vi "TestFGV.vi"() -> ()   [LabVIEW 2015]
uses:
  TypeDef/ActionEnum.ctl
panel:
  out "Flag Out 4":bool[](array[boolean])
  out "Flag Out 3":bool[](array[boolean])
  out "Flag Out 2":bool[](array[boolean])
  out "Flag Out":bool[](array[boolean])
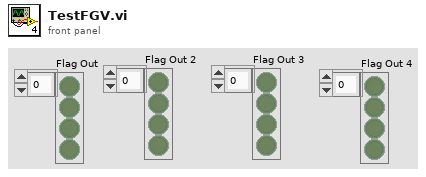
[diagram p1: front panel]
types:
  T1 = typedef "ActionEnum.ctl" = enum16{"Init", "Read", "Write"}
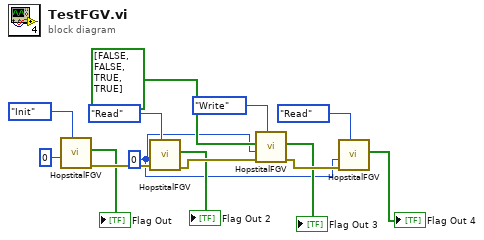
[diagram p0: block diagram]
diagram:
  w1 = 0 ("Room")
  n1 = call "HopstitalFGV.vi"(7:ActionEnum."Init", "Room"=0) -> ("error out"=w12:errorcluster, "Flag Out"=→"Flag Out":bool[])  [unwired: 8 in]
  n2 = call "HopstitalFGV.vi"(7:ActionEnum."Read", "error in (no error)"=w12, "Room"=w1) -> ("error out"=w11:errorcluster, "Flag Out"=→"Flag Out 2":bool[])  [unwired: 7 in]
  n3 = call "HopstitalFGV.vi"(7:ActionEnum."Write", "error in (no error)"=w11, "Room"=w1, "Flag In"=bool[] [FALSE, FALSE, TRUE, TRUE]) -> ("error out"=w10:errorcluster, "Flag Out"=→"Flag Out 3":bool[])  [unwired: 6 in]
  n4 = call "HopstitalFGV.vi"(7:ActionEnum."Read", "error in (no error)"=w10, "Room"=w1) -> ("Flag Out"=→"Flag Out 4":bool[])  [unwired: 7 in, 1 out]
